vi "CheckPolarityReversed.vi"(11 "3-phase current phase degrees":dbl[](array[numeric])) -> (3 "wiring information":string)   [LabVIEW 2017, in "McsaAnalysisLowRate.lvlib"]
uses:
  <vilib>/addons/InsightCM/Devices/Shared/Mcsa/McsaAnalysisLowRate/McsaAnalysisLowRate.lvlib
  <vilib>/Analysis/coordinate.llb/Angle Units.ctl
  <vilib>/Analysis/coordinate.llb/Angle Range (Degree).ctl
  <vilib>/Analysis/coordinate.llb/Wrap Angle (scalar).vi
  <vilib>/Analysis/NI_AAL_Angle.lvlib
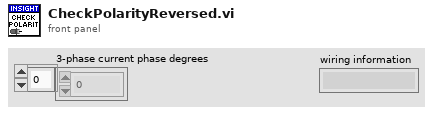
[diagram p1: front panel]
types:
  T1 = typedef "NI_AAL_Angle.lvlib/Angle Range (Degree).ctl" = u16
  T2 = typedef "NI_AAL_Angle.lvlib/Angle Units.ctl" = i32
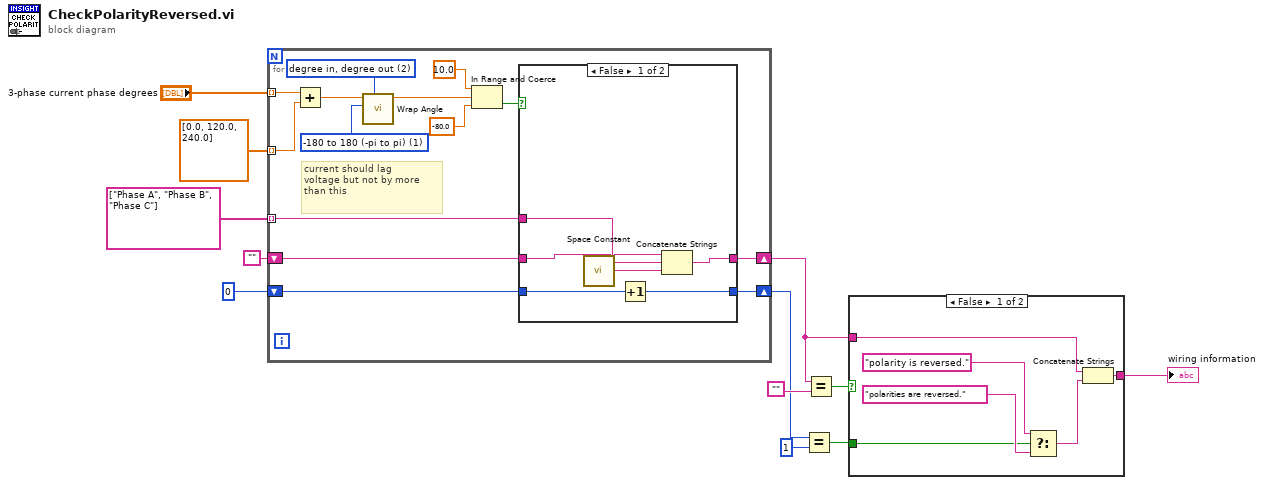
[diagram p0: block diagram]
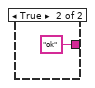
[diagram p2: hidden frame]
diagram:
  n1 = for {
    tunnel: "3-phase current phase degrees" -> [w26] mode=indexing
    tunnel: dbl[] [0.0, 120.0, 240.0] -> [w25] mode=indexing
    tunnel: string[] ["Phase A", "Phase B", "Phase C"] -> [w20] mode=indexing
    shift-right: [w21] -> w6
    shift-left: "" -> [w22]
    shift-right: [w18] -> w3
    shift-left: 0 -> [w17]
    w13 = T1 1 items=["none", "-180 to 180 (-pi to pi)", "0 to 360 (0 to 2pi)"] ("angle range")
    w14 = T2 2 items=["radian in, radian out", "radian in, degree out", "degree in, degree out", "degree in, radian out"] ("angle units")
    # "current should lag \nvoltage but not by more than this"
    n2 = Add(x=w26, y=w25) -> (x+y=w16:dbl)
    n3 = call-poly <vilib>:"Wrap Angle.vi"("angle units"=w14, "angle range"=w13, "angle in"=w16) -> ("angle out"=w15:dbl)  [unwired: 7 in, 1 out]
    n4 = In Range and Coerce(upper limit=10.0, x=w15, lower limit=-80.0) -> (In Range?=w19:bool)  [unwired: 1 out]
    n5 = case shown="False" w19 {
      tunnel: w22 -> [w30 w34]
      tunnel: [w32 w34] -> w21
      tunnel: w20 -> [w31 _]
      tunnel: [w28 w33] -> w18
      tunnel: w17 -> [w29 w33]
      frame False {
        n6 = call <vilib>:"Space Constant.vi"() -> ("String"=w27:string)
        n7 = Increment(x=w29) -> (x+1=w28:i32)
        n8 = Concatenate Strings(w30, w31, w27) -> (w32:string)
      }
      frame True {
        # "Correct wiring for this phase"
      }
    }
  }
  n9 = Equal?(x=w3, y=1) -> (x = y?=w4:bool)
  n10 = Equal?(x=w6, y="") -> (x = y?=w7:bool)
  n11 = case shown="False" w7 {
    tunnel: [w37 "ok"] -> w9
    tunnel: w4 -> [w35 _]
    tunnel: w6 -> [w36 _]
    frame False {
      n12 = Select(t="polarity is reversed.", s=w35, f="polarities are reversed.") -> (s? t:f=w38:string)
      n13 = Concatenate Strings(w36, w38) -> (w37:string)
    }
    frame True {
    }
  }
  "wiring information" <- w9
